vi "FT_Get_Modem_Status.vi"(0 "Handle":u32) -> (1 "FT_Status":u32(ring) items=["FT_OK", "FT_INVALID_HANDLE", "FT_DEVICE_NOT_FOUND", "FT_DEVICE_NOT_OPENED", "FT_IO_ERROR", "FT_INSUFFICIENT_RESOURCES", "FT_INVALID_PARAMETER", "FT_INVALID_BAUD_RATE", "FT_DEVICE_NOT_OPENED_FOR_ERASE", "FT_DEVICE_NOT_OPENED_FOR_WRITE", "FT_FAILED_TO_WRITE_DEVICE", "FT_EEPROM_READ_FAILED", "FT_EEPROM_WRITE_FAILED", "FT_EEPROM_ERASE_FAILED", "FT_EEPROM_NOT_PRESENT", "FT_EEPROM_NOT_PROGRAMMED", "FT_INVALID_ARGS", "FT_NOT_SUPPORTED", "FT_OTHER_ERROR"], 2 "Modem Status":T2, 3 "Line Status":T1)   [LabVIEW 2019, in "D2XX.lvlib"]
uses:
  D2XX.lvlib
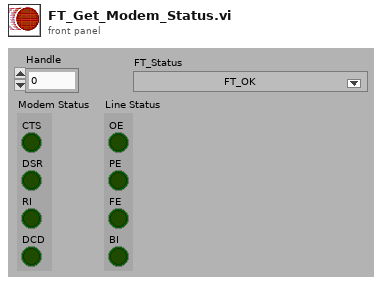
[diagram p1: front panel]
types:
  T1 = cluster{"OE":bool, "PE":bool, "FE":bool, "BI":bool}
  T2 = cluster{"CTS":bool, "DSR":bool, "RI":bool, "DCD":bool}
  T3 = cluster{"Boolean array[0]":bool, "Boolean array[1]":bool, "Boolean array[2]":bool, "Boolean array[3]":bool, "Boolean array[4]":bool, "Boolean array[5]":bool, "Boolean array[6]":bool, "Boolean array[7]":bool}
  T4 = cluster{"Boolean array[4]":bool, "Boolean array[5]":bool, "Boolean array[6]":bool, "Boolean array[7]":bool}
  T5 = cluster{"Boolean array[1]":bool, "Boolean array[2]":bool, "Boolean array[3]":bool, "Boolean array[4]":bool}
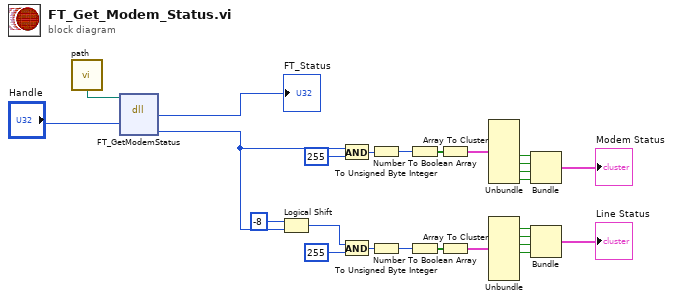
[diagram p0: block diagram]
diagram:
  n1 = call "path.vi"() -> ("lib path"=w1:path)
  n2 = dll-call lib="FTD2XX.dll" fn="FT_GetModemStatus"(path in=w1, "Handle"="Handle") -> (→"FT_Status":u32, "ModemStatus"=w13:u32)  [unwired: 4 in, 2 out]
  n3 = Logical Shift(y=-8, x=w13) -> (x << y=w11:u32)
  n4 = And(x=w13, y=u32 255) -> (x .and. y?=w23:u32)
  n5 = And(x=w11, y=u32 255) -> (x .and. y?=w7:u32)
  n6 = To Unsigned Byte Integer(number=w23) -> (unsigned 8bit integer=w20:u8)
  n7 = To Unsigned Byte Integer(number=w7) -> (unsigned 8bit integer=w8:u8)
  n8 = Number To Boolean Array(number=w20) -> (Boolean array=w22:bool[])
  n9 = Number To Boolean Array(number=w8) -> (Boolean array=w10:bool[])
  n10 = Array To Cluster(array=w22) -> (cluster=w21:T3)
  n11 = Array To Cluster(array=w10) -> (cluster=w9:T3)
  n12 = Unbundle(w21) -> ("Boolean array[4]"=w15:bool, "Boolean array[5]"=w16:bool, "Boolean array[6]"=w17:bool, "Boolean array[7]"=w18:bool)  [unwired: 4 out]
  n13 = Unbundle(w9) -> ("Boolean array[1]"=w6:bool, "Boolean array[2]"=w5:bool, "Boolean array[3]"=w4:bool, "Boolean array[4]"=w3:bool)  [unwired: 4 out]
  n14 = Bundle("Boolean array[4]"=w15, "Boolean array[5]"=w16, "Boolean array[6]"=w17, "Boolean array[7]"=w18) -> (→"Modem Status":T4)  [unwired: 1 in]
  n15 = Bundle("Boolean array[1]"=w6, "Boolean array[2]"=w5, "Boolean array[3]"=w4, "Boolean array[4]"=w3) -> (→"Line Status":T5)  [unwired: 1 in]
